vi "INI FILE READ.vi"(8 "error in (no error)":errorcluster, 11 "File Path":string="D:\\LAB-IQ 150\\WO 2476\\v01\\Data\\01_02_46_PM_02_July_2026\\01_02_46_PM_02_July_202601_02_46_PM_02_July_2026.csv") -> (0 "error out":errorcluster, 3 "concatenated string":string)   [LabVIEW 2025]
uses:
  Configuraton Files/Config file  FGV Unitest enum.ctl
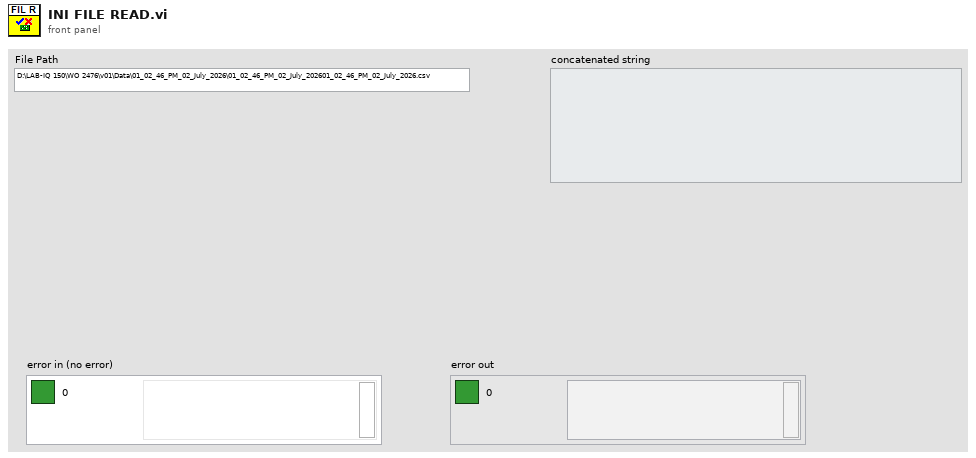
[diagram p1: front panel]
types:
  T1 = typedef "Config file  FGV Unitest enum.ctl" = enum16{"OPEN", "READ", "WRITE", "CLOSE"}
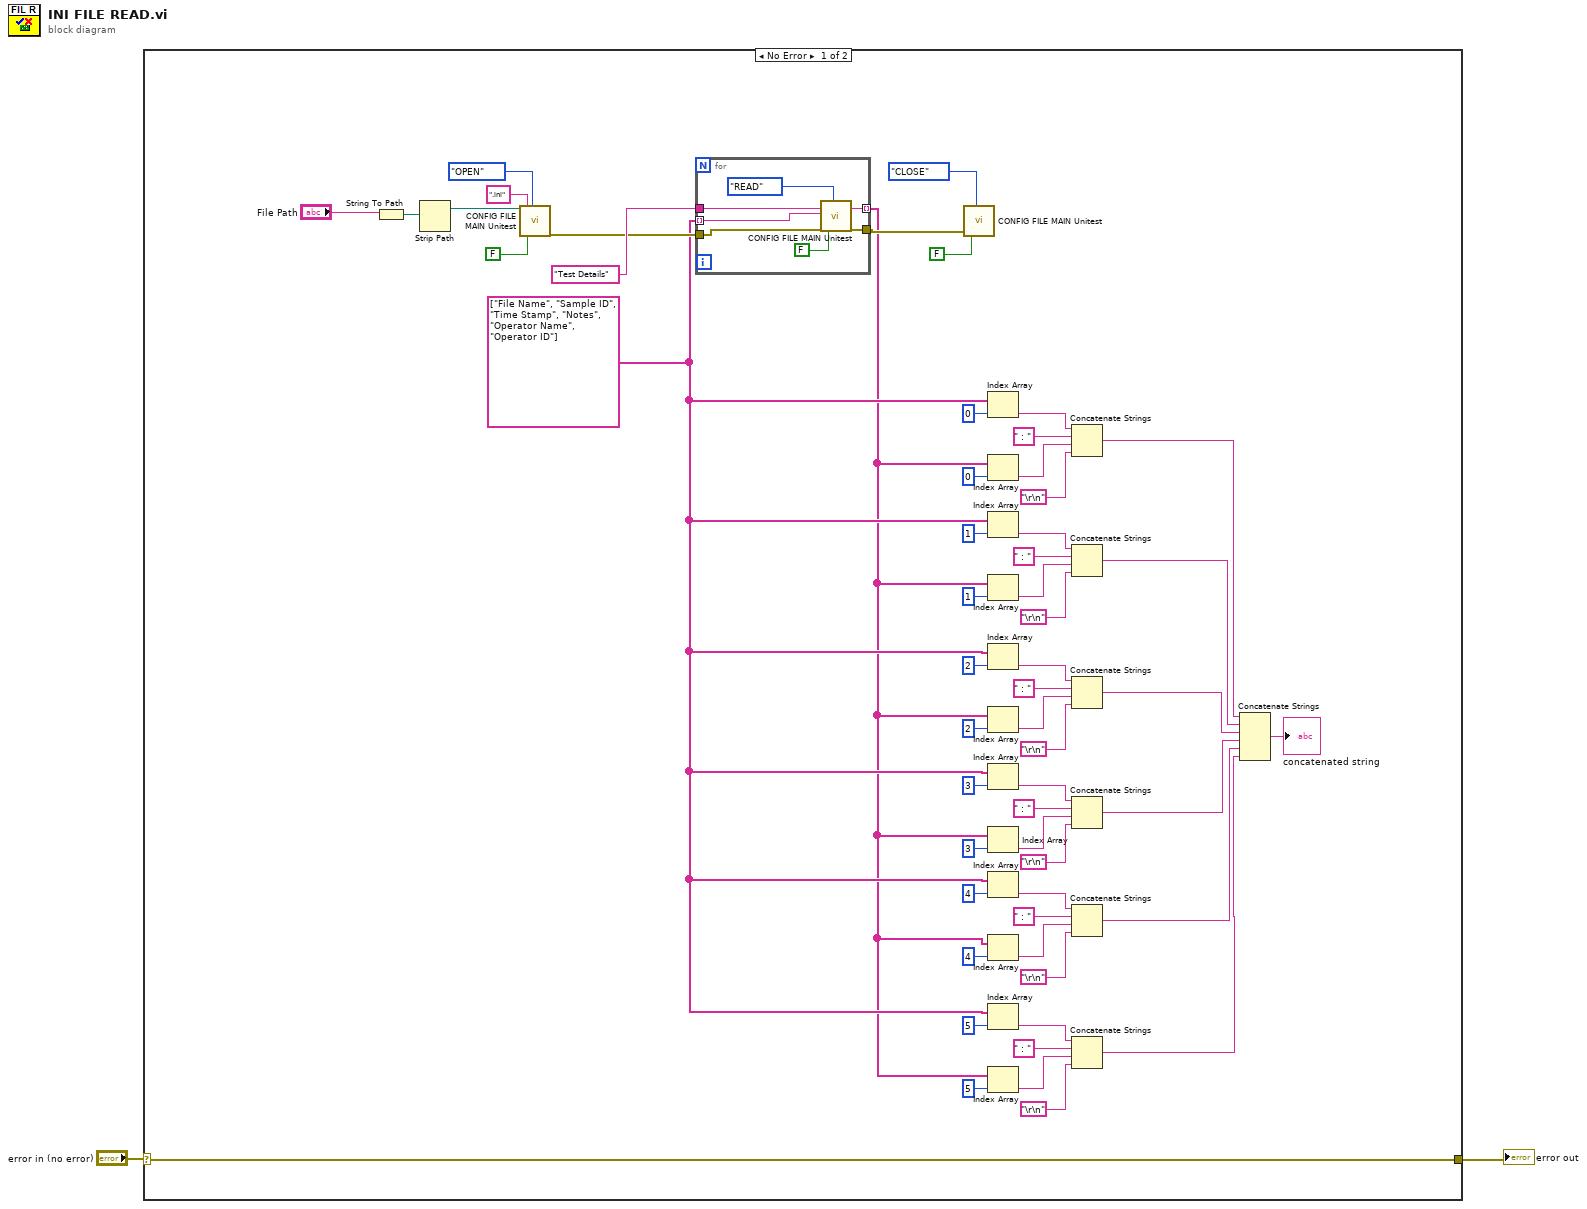
[diagram p0: block diagram]
diagram:
  n1 = case shown="No Error" "error in (no error)" {
    selector: "error in (no error)" -> [w3 _]
    tunnel: [w3 _] -> w1
    frame No Error {
      w12 = string[] ["File Name", "Sample ID", "Time Stamp", "Notes", "Operator Name", "Operator ID"] ("WRITE KEY")
      n2 = String To Path(string="File Path") -> (path=w59:path)
      n3 = Strip Path(path=w59) -> (stripped path=w49:path)  [unwired: 1 out]
      n4 = call "CONFIG FILE MAIN Unitest.vi"("File Path"=w49, "file name"=".ini", "PARAMETER/CONFIG"=FALSE, "Config Enum"=Config_file__FGV_Unitest_enum."OPEN") -> ("error out"=w53:errorcluster)  [unwired: 14 in, 1 out]
      n5 = for {
        tunnel: "Test Details" ("WRITE /READ SECTION") -> [w65]
        tunnel: [w64] -> w50
        tunnel: w12 -> [w62] mode=indexing
        tunnel: w53 -> [w61]
        tunnel: [w60] -> w11 mode=indexing
        n6 = call "CONFIG FILE MAIN Unitest.vi"("WRITE /READ SECTION"=w65, "READ KEY"=w62, "error in"=w61, "PARAMETER/CONFIG"=FALSE, "Config Enum"=Config_file__FGV_Unitest_enum."READ") -> ("READ VALUE"=w60:string, "error out"=w64:errorcluster)  [unwired: 13 in]
      }
      n7 = call "CONFIG FILE MAIN Unitest.vi"("error in"=w50, "PARAMETER/CONFIG"=FALSE, "Config Enum"=Config_file__FGV_Unitest_enum."CLOSE") -> ()  [unwired: 15 in, 2 out]
      n8 = Index Array(array=w12, index=0) -> (element=w48:string)
      n9 = Index Array(array=w11, index=0) -> (element=w47:string)
      n10 = Index Array(array=w12, index=1) -> (element=w37:string)
      n11 = Index Array(array=w11, index=1) -> (element=w38:string)
      n12 = Index Array(array=w12, index=2) -> (element=w31:string)
      n13 = Index Array(array=w11, index=2) -> (element=w32:string)
      n14 = Index Array(array=w12, index=3) -> (element=w30:string)
      n15 = Index Array(array=w11, index=3) -> (element=w29:string)
      n16 = Index Array(array=w12, index=4) -> (element=w19:string)
      n17 = Index Array(array=w11, index=4) -> (element=w20:string)
      n18 = Index Array(array=w12, index=5) -> (element=w13:string)
      n19 = Index Array(array=w11, index=5) -> (element=w14:string)
      n20 = Concatenate Strings(w48, " : " ("string"), w47, "\r\n") -> (w10:string)
      n21 = Concatenate Strings(w37, " : " ("string"), w38, "\r\n") -> (w9:string)
      n22 = Concatenate Strings(w31, " : " ("string"), w32, "\r\n") -> (w8:string)
      n23 = Concatenate Strings(w30, " : " ("string"), w29, "\r\n") -> (w7:string)
      n24 = Concatenate Strings(w19, " : " ("string"), w20, "\r\n") -> (w6:string)
      n25 = Concatenate Strings(w13, " : " ("string"), w14, "\r\n") -> (w5:string)
      n26 = Concatenate Strings(w10, w9, w8, w7, w6, w5) -> (→"concatenated string":string)
    }
    frame Error {
    }
  }
  "error out" <- w1
